vi "BoolCmd_ObtainQueue.vi"(11 "Command Name":string) -> (0 "error out":errorcluster, 3 "Queue out":refnum<queue>)   [LabVIEW 2019, in "Trajectory_Library.lvlib"]
uses:
  Trajectory_Library.lvlib
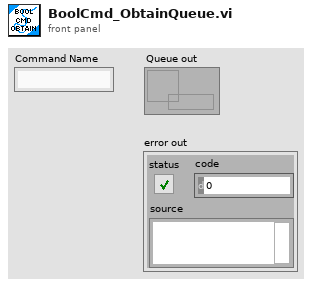
[diagram p1: front panel]
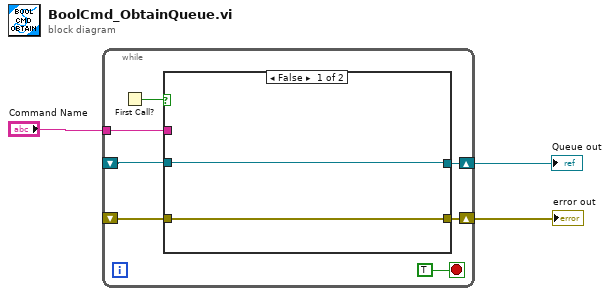
[diagram p0: block diagram]
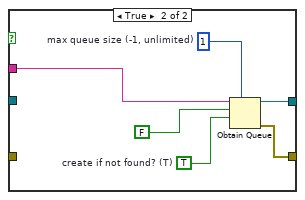
[diagram p2: hidden frame]
diagram:
  n1 = while {
    tunnel: "Command Name" -> [w10]
    shift-right: [w7] -> w3
    shift-left: _ -> [w6]
    shift-right: [w5] -> w1
    shift-left: _ -> [w4]
    stop <- TRUE stop-if-true
    n2 = First Call?() -> (First Call?: T/F=w8:bool)
    n3 = case shown="False" w8 {
      tunnel: w10 -> [_ w16]
      tunnel: [w12 w14] -> w7
      tunnel: w6 -> [w12 _]
      tunnel: [w11 w13] -> w5
      tunnel: w4 -> [w11 _]
      frame False {
      }
      frame True {
        w17 = TRUE  # create if not found? (T)
        w18 = 1  # max queue size (-1, unlimited)
        n4 = Obtain Queue(max queue size (-1, unlimited)=w18, name (unnamed)=w16, element data type=FALSE, create if not found? (T)=w17) -> (queue out=w14:refnum<queue>, error out=w13:errorcluster)  [unwired: 1 in, 1 out]
      }
    }
  }
  "Queue out" <- w3
  "error out" <- w1
